vi "SLL DE Create DAQmx task for given channels.vi"(7 "Channel Type":T1, 8 "error in (no error)":errorcluster, 9 "Number of elements":i32[](array[numeric]), 10 "Channel Names":string[][](array[string]), 11 "Found Device Names":string[](array[string])) -> (0 "error out":errorcluster, 3 "Array of Tasks":refnum<k21>[](array[refnum]))   [LabVIEW 2013]
doc: "Copyright © 2005, Soliton Technologies.\nAll rights reserved."
uses:
  Controls/SLL DE DAQ Engine Channel Types.ctl
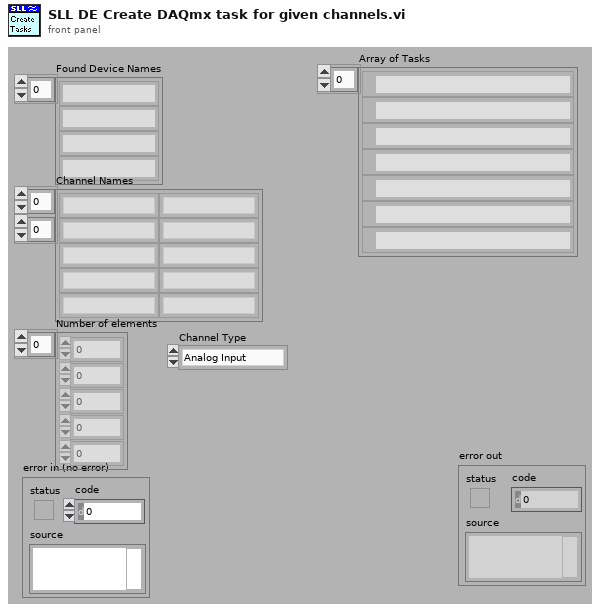
[diagram p1: front panel]
types:
  T1 = typedef "SLL DE DAQ Engine Channel Types.ctl" = enum16{"Analog Input", "Analog Output", "Digital Input", "Digital Output"}
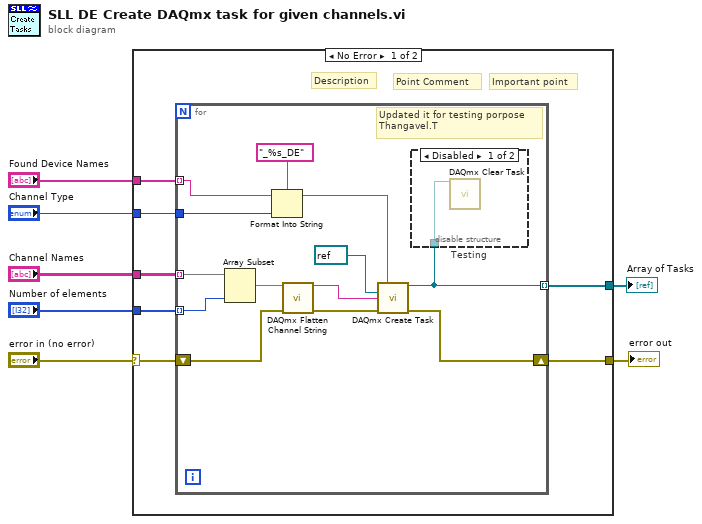
[diagram p0: block diagram]
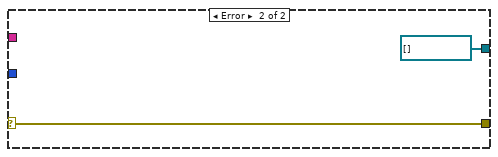
[diagram p3: hidden frame]
diagram:
  n1 = case shown="No Error" "error in (no error)" {
    selector: "error in (no error)" -> [w9 w30]
    tunnel: [w8 w30] -> w6
    tunnel: "Found Device Names" -> [w14 _]
    tunnel: "Channel Names" -> [w13 _]
    tunnel: "Number of elements" -> [w12 _]
    tunnel: "Channel Type" -> [w11 _]
    tunnel: [w10 refnum<k21>[] []] -> w1
    frame No Error {
      # "Point Comment"
      # "Important point"
      # "Description"
      n2 = for {
        tunnel: w14 -> [w20] mode=indexing
        tunnel: w13 -> [w27] mode=indexing
        tunnel: w12 -> [w26] mode=indexing
        shift-right: [w18] -> w8
        shift-left: w9 -> [w23]
        tunnel: w11 -> [w21]
        tunnel: [w16] -> w10 mode=indexing
        # "Updated it for testing porpose\nThangavel.T"
        n3 = Array Subset(array=w27, length=w26) -> (w25:string[])  [unwired: 1 in]
        n4 = Format Into String(format string="_%s_DE", initial string=w20, w21) -> (resulting string=w17:string)  [unwired: 1 in, 1 out]
        n5 = call <vilib>:"DAQmx Flatten Channel String.vi"("names in"=w25, "error in"=w23) -> ("names out"=w24:string, "error out"=w22:errorcluster)  [unwired: 12 in]
        n6 = call <vilib>:"DAQmx Create Task.vi"("new task name"=w17, "task to copy"=refnum<k21> refnum, "global virtual channels"=w24, "error in"=w22) -> ("task out"=w16:refnum<k21>, "error out"=w18:errorcluster)  [unwired: 10 in]
        n7 = disable-structure "Testing" shown="Disabled" {
          disable-tunnel: w16 -> [w28 _]
          frame Disabled {
            n8 = call <vilib>:"DAQmx Clear Task.vi"("task in"=w28) -> ()  [unwired: 14 in, 1 out]
          }
          frame Enabled {
          }
        }
      }
    }
    frame Error {
    }
  }
  "error out" <- w6
  "Array of Tasks" <- w1
